vi "captureTopBottomExp.vi"(8 "error in (no error)":errorcluster, 10 "Array in":refnum<k7>[](array[refnum]), 11 "Cluster in":refnum<vi>) -> (0 "error out":errorcluster, 3 "Value":T1)   [LabVIEW 2014]
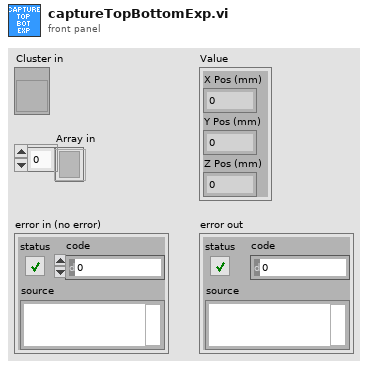
[diagram p1: front panel]
types:
  T1 = cluster{"X Pos (mm)":sgl, "Y Pos (mm)":sgl, "Z Pos (mm)":sgl}
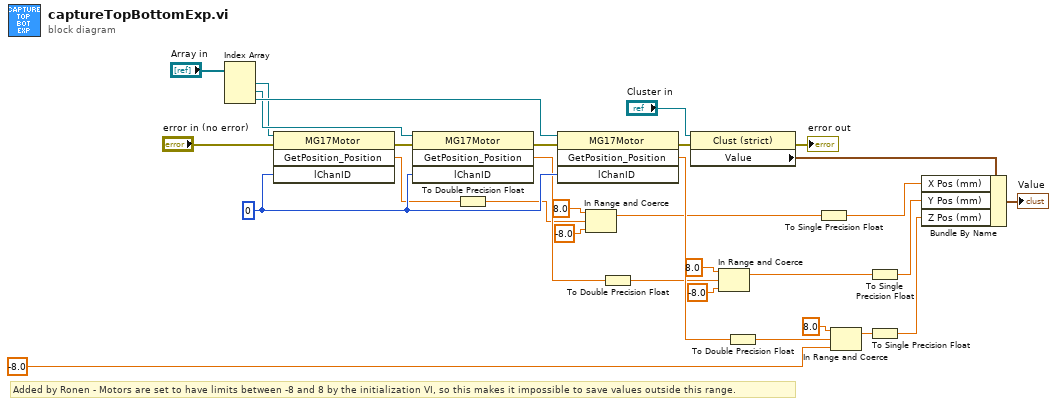
[diagram p0: block diagram]
diagram:
  w27 = 0 ("lChanID")
  # "Added by Ronen - Motors are set to have limits between -8 and 8 by the initialization VI, so this makes it impossible to save values outside this range."
  n1 = Index Array(array="Array in") -> (element #1=w21:refnum<k7>, element #2=w22:refnum<k7>, element #3=w23:refnum<k7>)  [unwired: 3 in]
  n2 = invoke class="MG17Motor" method="GetPosition_Position"(reference=w21, error in="error in (no error)", "lChanID"=w27) -> (error out=w30:errorcluster, "GetPosition_Position"=w8:sgl)  [unwired: 1 in, 2 out]
  n3 = invoke class="MG17Motor" method="GetPosition_Position"(reference=w22, error in=w30, "lChanID"=w27) -> (error out=w31:errorcluster, "GetPosition_Position"=w9:sgl)  [unwired: 1 in, 2 out]
  n4 = To Double Precision Float(number=w8) -> (double precision float=w7:dbl)
  n5 = invoke class="MG17Motor" method="GetPosition_Position"(reference=w23, error in=w31, "lChanID"=w27) -> (error out=w24:errorcluster, "GetPosition_Position"=w11:sgl)  [unwired: 1 in, 2 out]
  n6 = In Range and Coerce(upper limit=8.0, x=w7, lower limit=-8.0) -> (coerced(x)=w2:dbl)  [unwired: 1 out]
  n7 = To Double Precision Float(number=w9) -> (double precision float=w10:dbl)
  n8 = property on="Property Node" class="Clust (strict)"(reference="Cluster in", error in=w24) -> (error out=→"error out":errorcluster, "Value"=w25:T1)  [unwired: 1 out]
  n9 = In Range and Coerce(upper limit=8.0, x=w10, lower limit=-8.0) -> (coerced(x)=w4:dbl)  [unwired: 1 out]
  n10 = To Double Precision Float(number=w11) -> (double precision float=w12:dbl)
  n11 = To Single Precision Float(number=w2) -> (single precision float=w1:sgl)
  n12 = In Range and Coerce(upper limit=8.0, x=w12, lower limit=-8.0) -> (coerced(x)=w6:dbl)  [unwired: 1 out]
  n13 = To Single Precision Float(number=w4) -> (single precision float=w3:sgl)
  n14 = To Single Precision Float(number=w6) -> (single precision float=w5:sgl)
  n15 = Bundle By Name(cluster=w25, "X Pos (mm)"=w1, "Y Pos (mm)"=w3, "Z Pos (mm)"=w5) -> (→"Value":T1)
